vi "Begin.vi"(11 "Image Size":T1=enum."160x120") -> (0 "error out":errorcluster)   [LabVIEW 2012]
doc: "Called before other user functions, this VI is expected to open initial I/O refnums, load in file data, and do all program initialization. Notice that the <B>error out</B> terminal is simply used for data flow. Wiring it to other structures or subVIs ensures that this VI runs first."
uses:
  <vilib>/Rock Robotics/WPI/Camera/WPI_CameraImageSize.ctl
  <vilib>/Rock Robotics/WPI/Camera/WPI_CameraWhite Balance Values.ctl
  <vilib>/Rock Robotics/WPI/Camera/WPI_CameraExposure Values.ctl
  <vilib>/Rock Robotics/WPI/Camera/WPI_CameraFrameRate.ctl
  <vilib>/Rock Robotics/WPI/DriverStation/WPI_DriverStationRobotMode2.ctl
  <vilib>/Rock Robotics/WPI/Joystick/WPI_JoystickDeviceEnum.ctl
  <vilib>/Rock Robotics/SystemInterfaces/DIO/FPGA_DIOPWMChannel.ctl
  <vilib>/Rock Robotics/WPI/SafetyOutput/WPI_SafetyOutputConfigMenu.ctl
  <vilib>/Rock Robotics/SystemInterfaces/DIO/FPGA_DIORelayChannel.ctl
  <vilib>/Rock Robotics/SystemInterfaces/DIO/FPGA_DIOChannel.ctl
  <vilib>/Rock Robotics/WPI/Solenoid/WPI_SolenoidChannel.ctl
  Robot Global Data.vi
  <vilib>/Rock Robotics/WPI/RobotDrive/WPI_RobotDriveOpen4MotorWithJaguar.vi
  <vilib>/Rock Robotics/WPI/Solenoid/WPI_SolenoidOpenSingle.vi
  <vilib>/Rock Robotics/WPI/Compressor/WPI_CompressorGetSetRefNum.vi
  <vilib>/Rock Robotics/WPI/MotorControl/WPI_MotorControlOpen Jaguar.vi
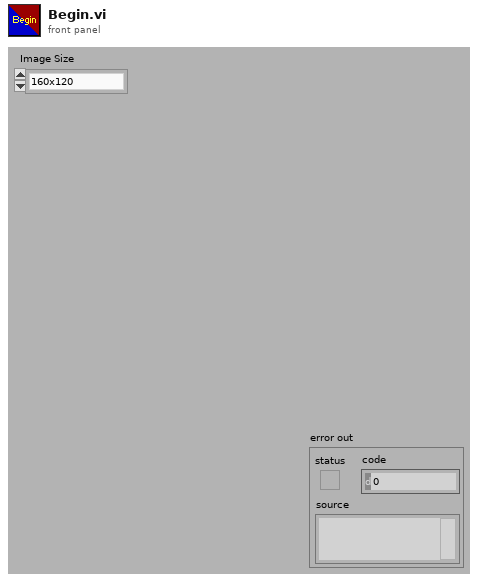
[diagram p1: front panel]
types:
  T1 = typedef "WPI_CameraImageSize.ctl" = enum16{"640x480", "320x240", "160x120"}
  T2 = typedef "WPI_JoystickDeviceEnum.ctl" = enum16{"USB 1", "USB 2", "USB 3", "USB 4", "Kinect 1", "Kinect 2"}
  T3 = typedef "WPI_SafetyOutputConfigMenu.ctl" = enum16{"Enable", "Disable"}
  T4 = typedef "FPGA_DIOPWMChannel.ctl" = enum8{"PWM 1", "PWM 2", "PWM 3", "PWM 4", "PWM 5", "PWM 6", "PWM 7", "PWM 8", "PWM 9", "PWM 10", "Invalid"}
  T5 = typedef "WPI_DriverStationRobotMode2.ctl" = enum16{"Autonomous Disabled", "Autonomous Enabled", "Teleop Disabled", "Teleop Enabled", "Timeout", "Finish", "Test Disabled", "Test Enabled"}
  T6 = typedef "WPI_CameraFrameRate.ctl" = u32
  T7 = typedef "WPI_CameraExposure Values.ctl" = enum16{"Auto", "Flicker-free 50 Hz", "Flicker-free 60 Hz", "Hold current"}
  T8 = typedef "WPI_CameraWhite Balance Values.ctl" = enum16{"Auto", "Fixed indoor", "Fixed outdoor 1", "Fixed outdoor 2", "Fixed fluorescent 1", "Fixed fluorescent 2", "Hold current"}
  T9 = typedef "WPI_SolenoidChannel.ctl" = enum8{"Solenoid 1", "Solenoid 2", "Solenoid 3", "Solenoid 4", "Solenoid 5", "Solenoid 6", "Solenoid 7", "Solenoid 8", "Invalid"}
  T10 = typedef "FPGA_DIOChannel.ctl" = enum8{"DIO 1", "DIO 2", "DIO 3", "DIO 4", "DIO 5", "DIO 6", "DIO 7", "DIO 8", "DIO 9", "DIO 10", "DIO 11", "DIO 12", "DIO 13", "DIO 14", "Invalid"}
  T11 = typedef "FPGA_DIORelayChannel.ctl" = enum8{"Relay 1", "Relay 2", "Relay 3", "Relay 4", "Relay 5", "Relay 6", "Relay 7", "Relay 8", "Invalid"}
  T12 = typedef "WPI_SolenoidDevRef.ctl" = cluster{"DevStatus":errorcluster, "Solenoid Module":T13, "Forward Solenoid Channel":T9, "Reverse Solenoid Channel":T9}
  T13 = typedef "FPGA_TypedefSolenoidModule.ctl" = enum16{"Solenoid Module 1", "Solenoid Module 2"}
  T14 = typedef "WPI_CompressorDevRef.ctl" = cluster{"DevStatus":errorcluster, "DigitalInputDevRef":T15, "RelayDevRef":T17}
  T15 = typedef "WPI_DigitalInputDevRef.ctl" = cluster{"DevStatus":errorcluster, "DIO Channel":T10, "Digital Module":T16}
  T16 = typedef "FPGA_TypedefDigitalModule.ctl" = enum16{"Digital Module 1", "Digital Module 2"}
  T17 = typedef "WPI_RelayDevRef.ctl" = cluster{"DevStatus":errorcluster, "Relay Channel":T11, "Digital Module":T16, "Relay Direction":T18}
  T18 = typedef "WPI_RelayDirection.ctl" = enum16{"Both directions", "Forward only", "Reverse only"}
  T19 = typedef "WPI_MotorControlDeviceRef.ctl" = cluster{"DeviceStatus":errorcluster, "Type":enum16{"PWM", "CAN"}, "PWM":cluster{"Digital Module":T16, "PWM Channel":T4, "DeadBand":T20}, "CAN":cluster{"Device Number":u8, "Control Mode":T21, "Semaphore":T22, "Max Vout":dbl}, "Invert":bool, "TransformRef":T23, "InvTransformRef":T23}
  T20 = typedef "WPI_PWMDeadband.ctl" = cluster{"Name":string, "maxPositivePwm":i32, "minPositivePwm":i32, "centerPwm":i32, "maxNegativePwm":i32, "minNegativePwm":i32, "angularRange":u16}
  T21 = typedef "WPI_CANJaguar_ControlMode.ctl" = enum8{"Percent VBus", "Current", "Speed", "Position", "Voltage"}
  T22 = typedef "Semaphore RefNum" = refnum<k1>
  T23 = typedef "WPI_PWMTransform_ConPane.ctl" = refnum<vi>
  T24 = typedef "FPGA_WatchdogDevRef.ctl" = cluster{"DevStatus":errorcluster}
  T25 = typedef "WPI_RobotDriveDevRef.ctl" = cluster{"DevStatus":errorcluster, "Motors[]":T19[], "Square Inputs":bool, "Max Output":dbl, "Isochronous":bool}
  T26 = typedef "WPI_JoystickDevRef.ctl" = cluster{"Device":T2}
  T27 = typedef "WPI_CameraDevRef.ctl" = cluster{"Camera Address":string, "CameraStatus":errorcluster, "Acquire Image Notifier":refnum<notifier>}
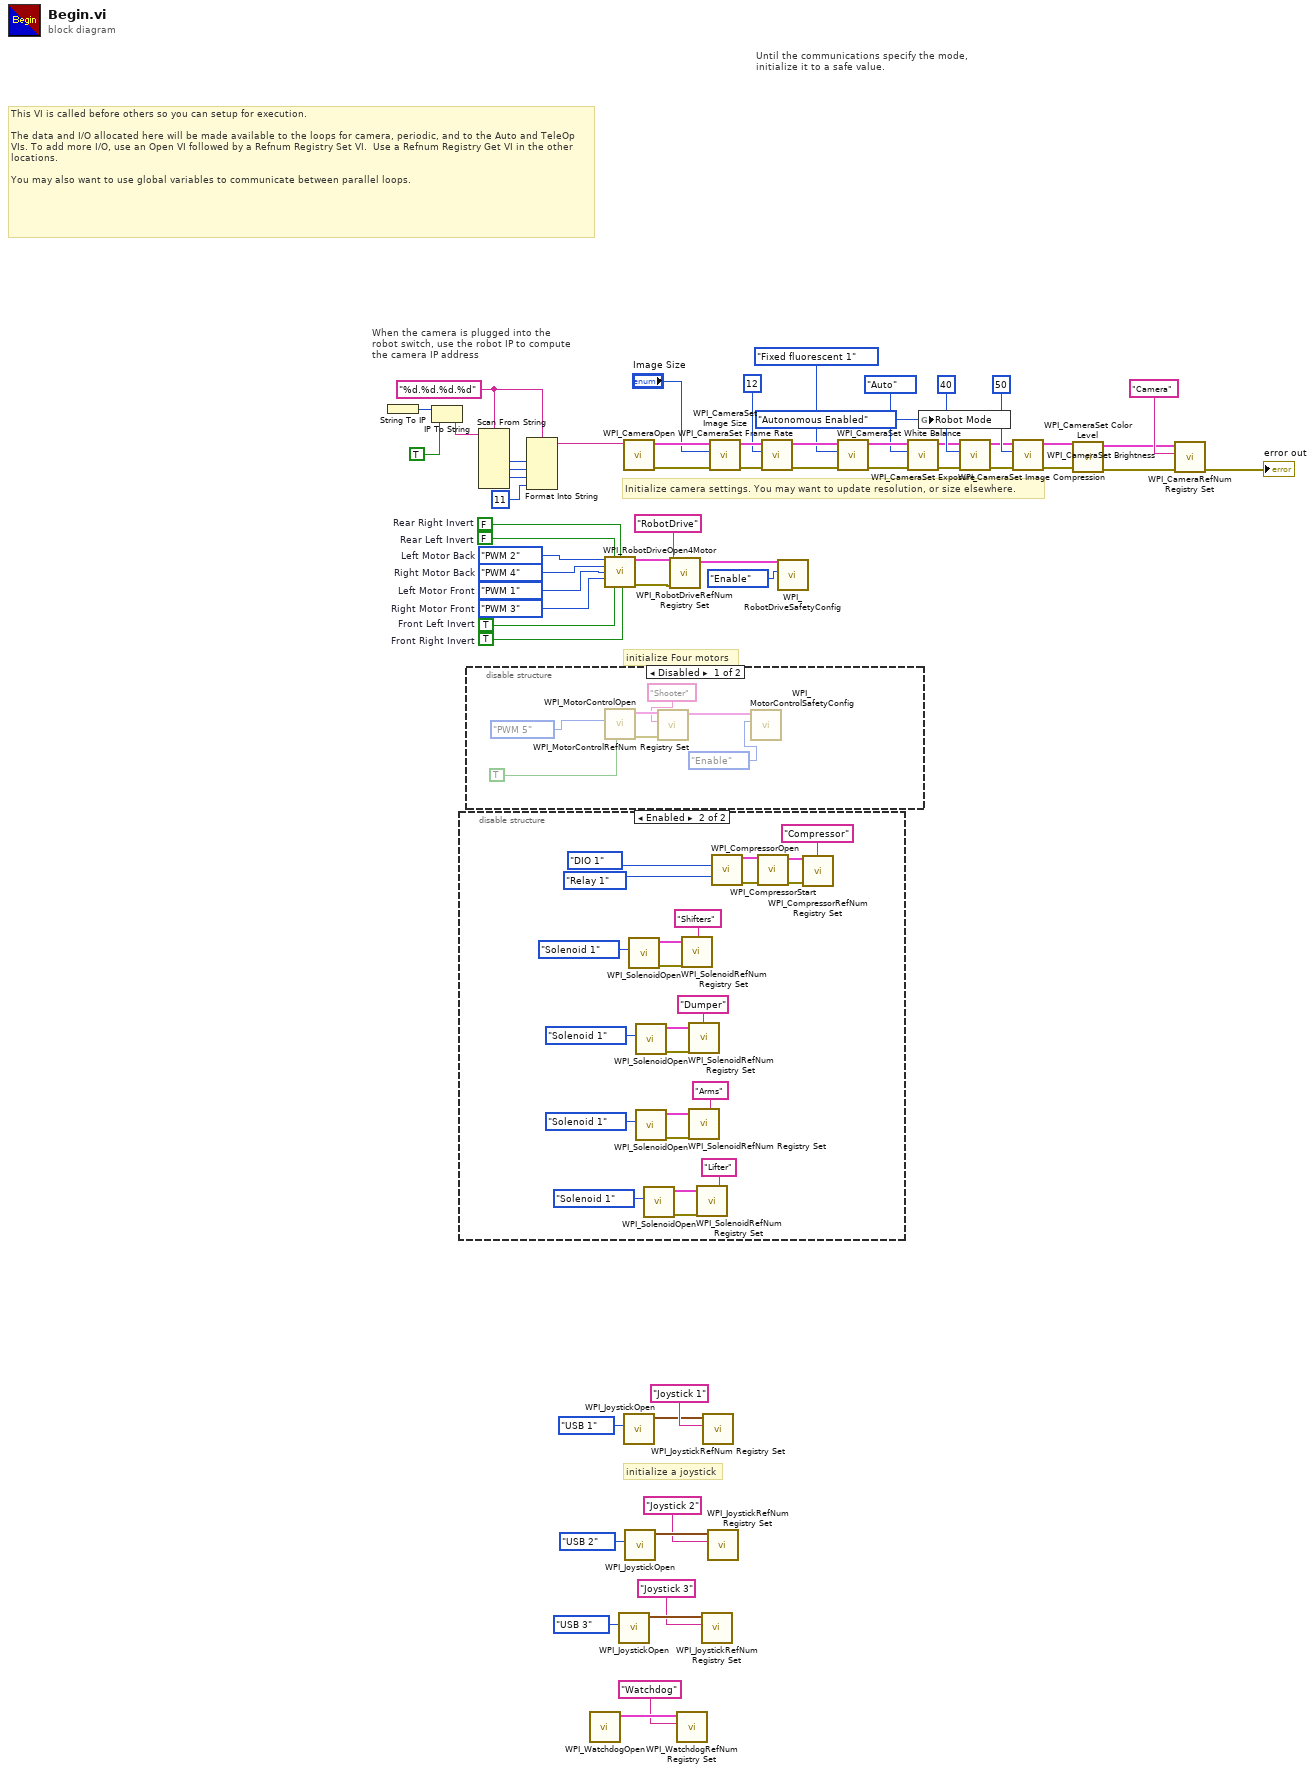
[diagram p0: block diagram]
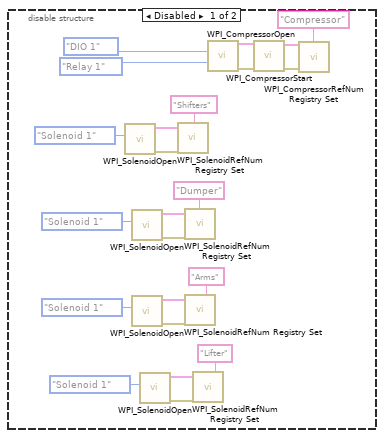
[diagram p2: hidden frame]
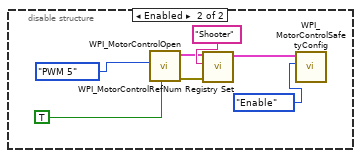
[diagram p3: hidden frame]
diagram:
  w13 = TRUE  # Front Right Invert
  w14 = TRUE  # Front Left Invert
  w19 = FPGA_DIOPWMChannel."PWM 4"  # Right Motor Back
  w16 = FPGA_DIOPWMChannel."PWM 3"  # Right Motor Front
  w18 = FPGA_DIOPWMChannel."PWM 2"  # Left Motor Back
  w17 = FPGA_DIOPWMChannel."PWM 1"  # Left Motor Front
  w12 = FALSE  # Rear Left Invert
  w15 = FALSE  # Rear Right Invert
  w32 = "%d.%d.%d.%d" ("format string")
  # "This VI is called before others so you can setup for execution.\n\nThe data and I/O allocated here will be made available to the loops for camera, periodic, and to the Auto and TeleOp VIs. To add more I/O, use an Open VI followed by a Refnum Registry Set VI.  Use a Refnum Registry Get VI in the other locations.\n\nYou may also want to use global variables to communicate between parallel loops."
  # "initialize a joystick"
  # "Until the communications specify the mode,\ninitialize it to a safe value."
  # "When the camera is plugged into the\nrobot switch, use the robot IP to compute\nthe camera IP address"
  # "initialize Four motors"
  # "Initialize camera settings. You may want to update resolution, or size elsewhere."
  n1 = String To IP() -> (0:w39:u32)  [unwired: 1 in]
  n2 = IP To String(1:TRUE ("dot notation? (F)"), 2:w39) -> (0:w37:string)
  n3 = disable-structure shown="Enabled" {
    frame Disabled {
      n4 = call-poly <vilib>:"WPI_SolenoidOpen.vi"("Solenoid Channel"=WPI_SolenoidChannel."Solenoid 1") -> ("error out"=w72:errorcluster, "SolenoidDevRef"=w73:T12)  [unwired: 9 in]
      n5 = call-poly <vilib>:"WPI_SolenoidOpen.vi"("Solenoid Channel"=WPI_SolenoidChannel."Solenoid 1") -> ("error out"=w68:errorcluster, "SolenoidDevRef"=w69:T12)  [unwired: 9 in]
      n6 = call-poly <vilib>:"WPI_SolenoidOpen.vi"("Solenoid Channel"=WPI_SolenoidChannel."Solenoid 1") -> ("error out"=w64:errorcluster, "SolenoidDevRef"=w65:T12)  [unwired: 9 in]
      n7 = call-poly <vilib>:"WPI_SolenoidOpen.vi"("Solenoid Channel"=WPI_SolenoidChannel."Solenoid 1") -> ("error out"=w60:errorcluster, "SolenoidDevRef"=w61:T12)  [unwired: 9 in]
      n8 = call <vilib>:"WPI_SolenoidRefNum Registry Set.vi"("error in (no error)"=w72, "refnum name"="Shifters", "SolenoidDevRef"=w73) -> ()  [unwired: 7 in, 2 out]
      n9 = call <vilib>:"WPI_SolenoidRefNum Registry Set.vi"("error in (no error)"=w68, "refnum name"="Dumper", "SolenoidDevRef"=w69) -> ()  [unwired: 7 in, 2 out]
      n10 = call <vilib>:"WPI_SolenoidRefNum Registry Set.vi"("error in (no error)"=w64, "refnum name"="Arms", "SolenoidDevRef"=w65) -> ()  [unwired: 7 in, 2 out]
      n11 = call <vilib>:"WPI_SolenoidRefNum Registry Set.vi"("error in (no error)"=w60, "refnum name"="Lifter", "SolenoidDevRef"=w61) -> ()  [unwired: 7 in, 2 out]
      n12 = call <vilib>:"WPI_CompressorOpen.vi"("Pressure Switch DIO Channel"=FPGA_DIOChannel."DIO 1", "Relay Channel"=FPGA_DIORelayChannel."Relay 1") -> ("CompressorDevRef"=w78:T14, "error out"=w79:errorcluster)  [unwired: 12 in]
      n13 = call <vilib>:"WPI_CompressorStart.vi"("error in (no error)"=w79, "CompressorDevRef"=w78) -> ("error out"=w76:errorcluster, "CompressorDevRef"=w77:T14)  [unwired: 8 in]
      n14 = call <vilib>:"WPI_CompressorRefNum Registry Set.vi"("error in (no error)"=w76, "refnum name"="Compressor", "CompressorDevRef"=w77) -> ()  [unwired: 7 in, 2 out]
    }
    frame Enabled {
      n15 = call-poly <vilib>:"WPI_SolenoidOpen.vi"("Solenoid Channel"=WPI_SolenoidChannel."Solenoid 1") -> ("error out"=w91:errorcluster, "SolenoidDevRef"=w90:T12)  [unwired: 9 in]
      n16 = call-poly <vilib>:"WPI_SolenoidOpen.vi"("Solenoid Channel"=WPI_SolenoidChannel."Solenoid 1") -> ("error out"=w95:errorcluster, "SolenoidDevRef"=w94:T12)  [unwired: 9 in]
      n17 = call-poly <vilib>:"WPI_SolenoidOpen.vi"("Solenoid Channel"=WPI_SolenoidChannel."Solenoid 1") -> ("error out"=w99:errorcluster, "SolenoidDevRef"=w98:T12)  [unwired: 9 in]
      n18 = call-poly <vilib>:"WPI_SolenoidOpen.vi"("Solenoid Channel"=WPI_SolenoidChannel."Solenoid 1") -> ("error out"=w103:errorcluster, "SolenoidDevRef"=w102:T12)  [unwired: 9 in]
      n19 = call <vilib>:"WPI_SolenoidRefNum Registry Set.vi"("error in (no error)"=w91, "refnum name"="Shifters", "SolenoidDevRef"=w90) -> ()  [unwired: 7 in, 2 out]
      n20 = call <vilib>:"WPI_SolenoidRefNum Registry Set.vi"("error in (no error)"=w95, "refnum name"="Dumper", "SolenoidDevRef"=w94) -> ()  [unwired: 7 in, 2 out]
      n21 = call <vilib>:"WPI_SolenoidRefNum Registry Set.vi"("error in (no error)"=w99, "refnum name"="Arms", "SolenoidDevRef"=w98) -> ()  [unwired: 7 in, 2 out]
      n22 = call <vilib>:"WPI_SolenoidRefNum Registry Set.vi"("error in (no error)"=w103, "refnum name"="Lifter", "SolenoidDevRef"=w102) -> ()  [unwired: 7 in, 2 out]
      n23 = call <vilib>:"WPI_CompressorOpen.vi"("Pressure Switch DIO Channel"=FPGA_DIOChannel."DIO 1", "Relay Channel"=FPGA_DIORelayChannel."Relay 1") -> ("CompressorDevRef"=w85:T14, "error out"=w84:errorcluster)  [unwired: 12 in]
      n24 = call <vilib>:"WPI_CompressorStart.vi"("error in (no error)"=w84, "CompressorDevRef"=w85) -> ("error out"=w87:errorcluster, "CompressorDevRef"=w86:T14)  [unwired: 8 in]
      n25 = call <vilib>:"WPI_CompressorRefNum Registry Set.vi"("error in (no error)"=w87, "refnum name"="Compressor", "CompressorDevRef"=w86) -> ()  [unwired: 7 in, 2 out]
    }
  }
  n26 = disable-structure shown="Disabled" {
    frame Disabled {
      n27 = call-poly <vilib>:"WPI_MotorControlOpen.vi"("Invert"=TRUE, "PWM Channel"=FPGA_DIOPWMChannel."PWM 5") -> ("error out"=w110:errorcluster, "MotorControlDeviceRef"=w109:T19)  [unwired: 8 in]
      n28 = call <vilib>:"WPI_MotorControlRefNum Registry Set.vi"("error in (no error)"=w110, "refnum name"="Shooter", "MotorControlDevRef"=w109) -> ("MotorControlDevRef"=w111:T19)  [unwired: 7 in, 1 out]
      n29 = call <vilib>:"WPI_MotorControlSafetyConfig.vi"("mode"=WPI_SafetyOutputConfigMenu."Enable", "MotorControlDevRef"=w111) -> ()  [unwired: 8 in, 2 out]
    }
    frame Enabled {
      n30 = call-poly <vilib>:"WPI_MotorControlOpen.vi"("Invert"=TRUE, "PWM Channel"=FPGA_DIOPWMChannel."PWM 5") -> ("error out"=w113:errorcluster, "MotorControlDeviceRef"=w114:T19)  [unwired: 8 in]
      n31 = call <vilib>:"WPI_MotorControlRefNum Registry Set.vi"("error in (no error)"=w113, "refnum name"="Shooter", "MotorControlDevRef"=w114) -> ("MotorControlDevRef"=w112:T19)  [unwired: 7 in, 1 out]
      n32 = call <vilib>:"WPI_MotorControlSafetyConfig.vi"("mode"=WPI_SafetyOutputConfigMenu."Enable", "MotorControlDevRef"=w112) -> ()  [unwired: 8 in, 2 out]
    }
  }
  n33 = Scan From String(format string=w32, input string=w37) -> (output 1=w36:i32, output 2=w35:i32, output 3=w34:i32)  [unwired: 7 in, 3 out]
  n34 = Format Into String(format string=w32, w36, w35, w34, 11 ("Compression")) -> (resulting string=w31:string)  [unwired: 2 in, 1 out]
  n35 = call <vilib>:"WPI_WatchdogOpen.vi"() -> ("WatchdogDevRef"=w2:T24)  [unwired: 10 in, 1 out]
  n36 = call-poly <vilib>:"WPI_RobotDriveOpen4Motor.vi"("Rear Left Motor"=w18, "Rear Left Motor Inverted"=w12, "Rear Right Motor Inverted"=w15, "Rear Right Motor"=w19, "Front Left Motor"=w17, "Front Right Motor"=w16, "Front Left Motor Inverted"=w14, "Front Right Motor Inverted"=w13) -> ("RobotDriveDevRef"=w11:T25, "error out"=w10:errorcluster)  [unwired: 6 in]
  n37 = call <vilib>:"WPI_JoystickOpen.vi"("JoystickDevice"=WPI_JoystickDeviceEnum."USB 3") -> ("JoystickDevRef"=w4:T26)  [unwired: 10 in]
  n38 = call <vilib>:"WPI_CameraOpen.vi"("Camera Address"=w31) -> ("error out"=w49:errorcluster, "CameraDevRef"=w50:T27)  [unwired: 2 in, 7 out]
  n39 = call <vilib>:"WPI_JoystickOpen.vi"("JoystickDevice"=WPI_JoystickDeviceEnum."USB 1") -> ("JoystickDevRef"=w29:T26)  [unwired: 10 in]
  n40 = call <vilib>:"WPI_JoystickOpen.vi"("JoystickDevice"=WPI_JoystickDeviceEnum."USB 2") -> ("JoystickDevRef"=w25:T26)  [unwired: 10 in]
  n41 = call <vilib>:"WPI_RobotDriveRefNum Registry Set.vi"("error in (no error)"=w10, "refnum name"="RobotDrive", "RobotDriveDevRef"=w11) -> ("RobotDriveDevRef"=w8:T25)  [unwired: 8 out]
  n42 = call <vilib>:"WPI_WatchdogRefNum Registry Set.vi"("refnum name"="Watchdog", "WatchdogDevRef"=w2) -> ()  [unwired: 8 in, 2 out]
  n43 = call <vilib>:"WPI_JoystickRefNum Registry Set.vi"("refnum name"="Joystick 3", "JoystickDevRef"=w4) -> ()  [unwired: 8 in, 2 out]
  n44 = call <vilib>:"WPI_JoystickRefNum Registry Set.vi"("refnum name"="Joystick 1", "JoystickDevRef"=w29) -> ()  [unwired: 8 in, 2 out]
  n45 = call <vilib>:"WPI_JoystickRefNum Registry Set.vi"("refnum name"="Joystick 2", "JoystickDevRef"=w25) -> ()  [unwired: 8 in, 2 out]
  n46 = call <vilib>:"WPI_CameraSet Image Size.vi"("error in (no error)"=w49, "Image Size"="Image Size", "CameraDevRef"=w50) -> ("error out"=w48:errorcluster, "CameraDevRef Out"=w51:T27)  [unwired: 7 out]
  n47 = call <vilib>:"WPI_CameraSet Frame Rate.vi"("error in (no error)"=w48, "Frame Rate (fps)"=T6 12, "CameraDevRef"=w51) -> ("error out"=w47:errorcluster, "CameraDevRef Out"=w53:T27)  [unwired: 7 out]
  n48 = call <vilib>:"WPI_RobotDriveSafetyConfig.vi"("mode"=WPI_SafetyOutputConfigMenu."Enable", "RobotDriveDevRef"=w8) -> ()  [unwired: 8 in, 2 out]
  n49 = call <vilib>:"WPI_CameraSet White Balance.vi"("error in (no error)"=w47, "White Balance"=WPI_CameraWhite_Balance_Values."Fixed fluorescent 1", "CameraDevRef"=w53) -> ("error out"=w46:errorcluster, "CameraDevRef Out"=w52:T27)  [unwired: 7 out]
  n50 = call <vilib>:"WPI_CameraSet Exposure.vi"("error in (no error)"=w46, "Exposure"=WPI_CameraExposure_Values."Auto", "CameraDevRef"=w52) -> ("error out"=w45:errorcluster, "CameraDevRef Out"=w55:T27)  [unwired: 7 out]
  n51 = global write "Robot Global Data.vi" "Robot Mode"(WPI_DriverStationRobotMode2."Autonomous Enabled" ("Robot Mode")) -> ()
  n52 = call <vilib>:"WPI_CameraSet Image Compression.vi"("error in (no error)"=w45, "Compression"=40, "CameraDevRef"=w55) -> ("error out"=w44:errorcluster, "CameraDevRef Out"=w54:T27)  [unwired: 7 out]
  n53 = call <vilib>:"WPI_CameraSet Brightness.vi"("error in (no error)"=w44, "Brightness"=50, "CameraDevRef"=w54) -> ("error out"=w23:errorcluster, "CameraDevRef Out"=w22:T27)  [unwired: 7 out]
  n54 = call <vilib>:"WPI_CameraSet Color Level.vi"("error in (no error)"=w23, "CameraDevRef"=w22) -> ("error out"=w20:errorcluster, "CameraDevRef Out"=w21:T27)  [unwired: 8 in]
  n55 = call <vilib>:"WPI_CameraRefNum Registry Set.vi"("error in (no error)"=w20, "refnum name"="Camera", "CameraDevRef"=w21) -> ("error out"=→"error out":errorcluster)  [unwired: 8 out]
